vi "led.vi"() -> ()   [LabVIEW 2023]
uses:
  <vilib>/regexp/Match Regular Expression.xnode
panel:
  in  "Off":bool
  out "error out":errorcluster
  in  "error in":errorcluster
  in  "Stop":bool
  in  "LED input":string
  in  "On":bool
  out "LED 10":bool
  out "LED 9":bool
  out "LED 8":bool
  out "LED 7":bool
  out "LED 6":bool
  out "LED 5":bool
  out "LED 4":bool
  out "LED 3":bool
  out "LED 2":bool
  out "LED 1":bool
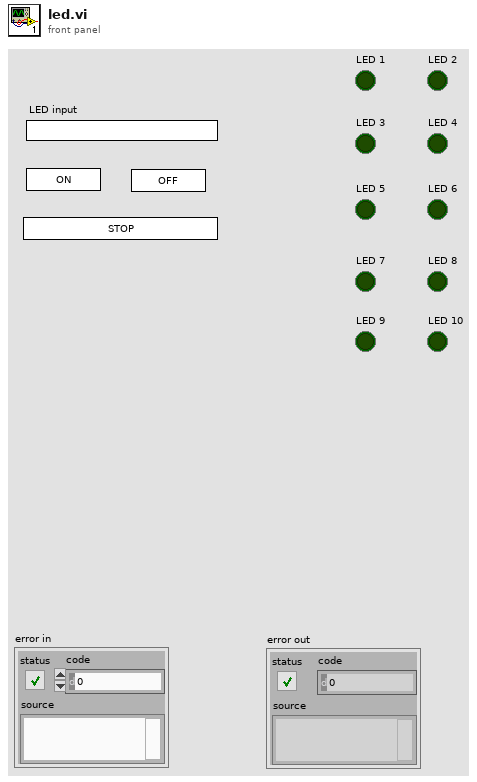
[diagram p1: front panel]
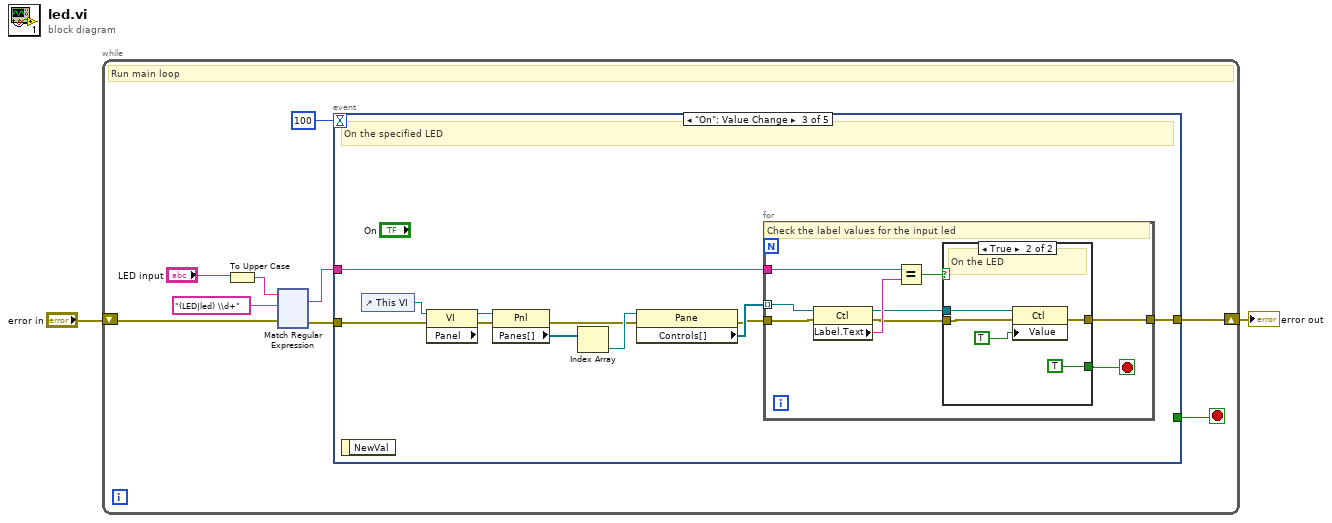
[diagram p0: block diagram]
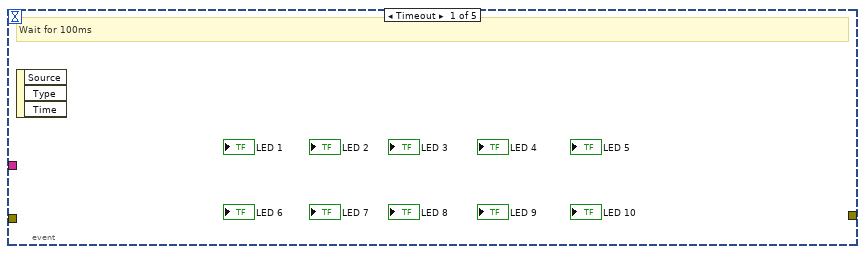
[diagram p2: hidden frame]
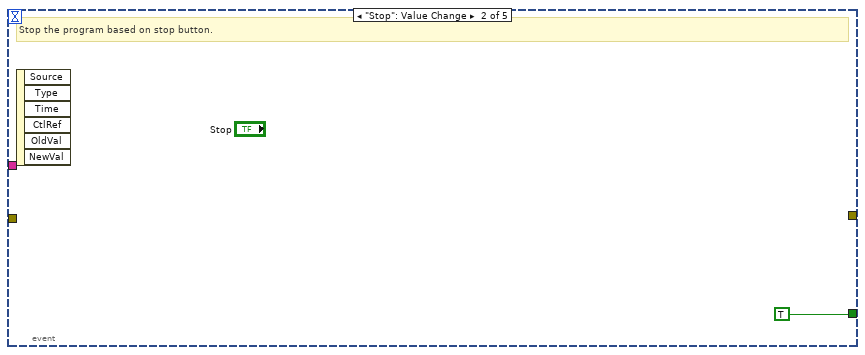
[diagram p3: hidden frame]
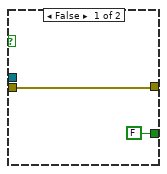
[diagram p4: hidden frame]
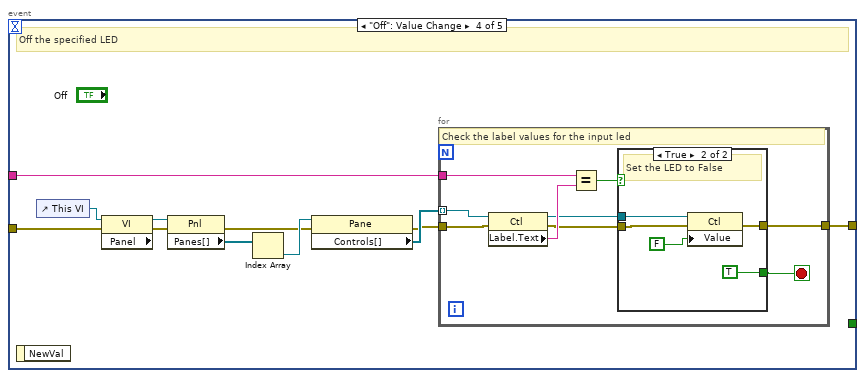
[diagram p5: hidden frame]
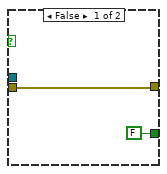
[diagram p6: hidden frame]
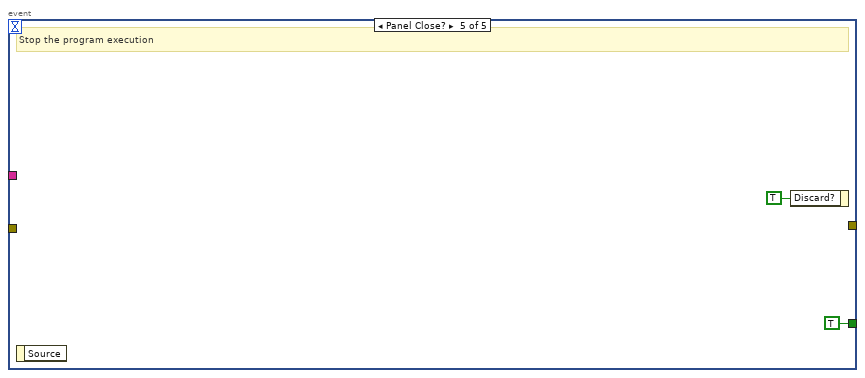
[diagram p7: hidden frame]
diagram:
  n1 = while {
    shift-right: [w3] -> w1
    shift-left: "error in" -> [w5]
    stop <- w9 stop-if-true
    # "Run main loop"
    n2 = To Upper Case(1:"LED input") -> (0:w8:string)
    n3 = xnode "Match Regular Expression"("input string"=w8, "regular expression"="(LED|led) \\d+", "error in"=w5) -> ("whole match"=w6:string, "error out"=w4:errorcluster)  [unwired: 3 in, 3 out]
    n4 = event shown="[2] \"On\": Value Change" {
      selector: _ -> [_ _ _ _ _]
      dyn-events: _ -> [_ _ _ _ _]
      timeout: 100 -> [_ _ _ _ _]
      tunnel: [_ TRUE _ _ TRUE] -> w9
      tunnel: w6 -> [_ _ w135 w161 _]
      tunnel: w4 -> [_ _ w134 w160 _]
      tunnel: [_ _ w130 w156 _] -> w3
      event Timeout {
        # "Wait for 100ms"
        n5 = event-data() -> ()  [unwired: 1 in, 3 out]
      }
      event "Stop": Value Change {
        # "Stop the program based on stop button."
        n6 = event-data() -> ()  [unwired: 1 in, 6 out]
      }
      event "On": Value Change {
        # "On the specified LED"
        n7 = event-data() -> ()  [unwired: 1 in, 1 out]
        n8 = control-ref of="This VI"() -> (w140:refnum<vi>)
        n9 = property class="VI"(reference=w140, error in=w134) -> (error out=w133:errorcluster, "Panel"=w139:refnum<vi>)  [unwired: 1 out]
        n10 = property class="Pnl"(reference=w139, error in=w133) -> (error out=w132:errorcluster, "Panes[]"=w138:refnum<vi>[])  [unwired: 1 out]
        n11 = Index Array(array=w138) -> (element=w137:refnum<vi>)  [unwired: 1 in]
        n12 = property class="Pane"(reference=w137, error in=w132) -> (error out=w131:errorcluster, "Controls[]"=w136:refnum<vi>[])  [unwired: 1 out]
        n13 = for {
          tunnel: w136 -> [w146] mode=indexing
          tunnel: w135 -> [w145]
          tunnel: w131 -> [w144]
          tunnel: [w142] -> w130
          stop <- w141 stop-if-true
          # "Check the label values for the input led"
          n14 = property class="Ctl"(reference=w146, error in=w144) -> (error out=w143:errorcluster, "Label.Text"=w148:string)  [unwired: 1 out]
          n15 = Equal?(x=w145, y=w148) -> (x = y?=w147:bool)
          n16 = case shown="True" w147 {
            tunnel: w146 -> [_ w155]
            tunnel: w143 -> [w150 w153]
            tunnel: [w150 w152] -> w142
            tunnel: [FALSE TRUE] -> w141
            frame False {
            }
            frame True {
              # "On the LED"
              n17 = property class="Ctl"(reference=w155, error in=w153, "Value"=TRUE) -> (error out=w152:errorcluster)  [unwired: 1 out]
            }
          }
        }
      }
      event "Off": Value Change {
        # "Off the specified LED"
        n18 = event-data() -> ()  [unwired: 1 in, 1 out]
        n19 = control-ref of="This VI"() -> (w166:refnum<vi>)
        n20 = property class="VI"(reference=w166, error in=w160) -> (error out=w159:errorcluster, "Panel"=w165:refnum<vi>)  [unwired: 1 out]
        n21 = property class="Pnl"(reference=w165, error in=w159) -> (error out=w158:errorcluster, "Panes[]"=w164:refnum<vi>[])  [unwired: 1 out]
        n22 = Index Array(array=w164) -> (element=w163:refnum<vi>)  [unwired: 1 in]
        n23 = property class="Pane"(reference=w163, error in=w158) -> (error out=w157:errorcluster, "Controls[]"=w162:refnum<vi>[])  [unwired: 1 out]
        n24 = for {
          tunnel: w162 -> [w172] mode=indexing
          tunnel: w161 -> [w171]
          tunnel: w157 -> [w170]
          tunnel: [w168] -> w156
          stop <- w167 stop-if-true
          # "Check the label values for the input led"
          n25 = property class="Ctl"(reference=w172, error in=w170) -> (error out=w169:errorcluster, "Label.Text"=w174:string)  [unwired: 1 out]
          n26 = Equal?(x=w171, y=w174) -> (x = y?=w173:bool)
          n27 = case shown="True" w173 {
            tunnel: w172 -> [_ w181]
            tunnel: w169 -> [w176 w179]
            tunnel: [w176 w178] -> w168
            tunnel: [FALSE TRUE] -> w167
            frame False {
            }
            frame True {
              # "Set the LED to False"
              n28 = property class="Ctl"(reference=w181, error in=w179, "Value"=FALSE) -> (error out=w178:errorcluster)  [unwired: 1 out]
            }
          }
        }
      }
      event Panel Close? {
        # "Stop the program execution"
        n29 = event-data() -> ()  [unwired: 1 in, 1 out]
        n30 = event-data("Discard?"=TRUE) -> ()  [unwired: 1 in, 1 out]
      }
    }
  }
  "error out" <- w1
